vi "Read hostname.vi"(8 "error in":errorcluster, 11 "PL_Target Configuration in":refnum<class "PL_Target Configuration.lvclass">) -> (0 "error out":errorcluster, 2 "hostname":string, 3 "PL_Target Configuration out":refnum<class "PL_Target Configuration.lvclass">)   [LabVIEW 2013, in "PL_Target Configuration.lvclass"]
uses:
  PL_Target Configuration.lvclass
  PL_Target Configuration.lvclass/PL_Target Configuration.ctl
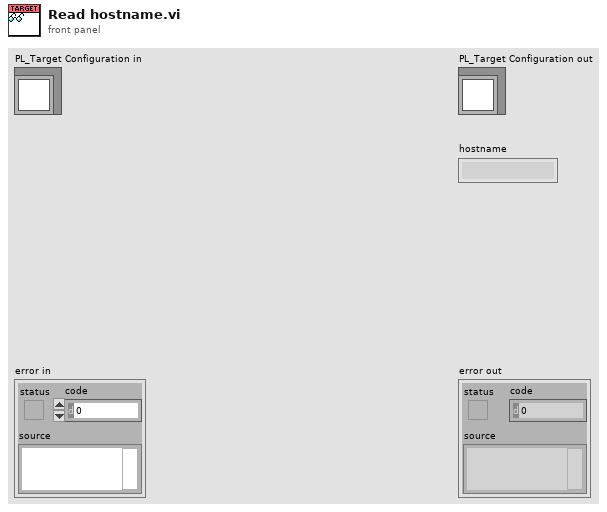
[diagram p1: front panel]
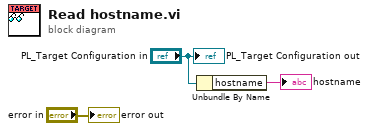
[diagram p0: block diagram]
diagram:
  n1 = Unbundle By Name("PL_Target Configuration in") -> ("hostname"=→"hostname":string)
  "error out" <- "error in"
  "PL_Target Configuration out" <- "PL_Target Configuration in"
